vi "Control Arm Gripper.vi"() -> ()   [LabVIEW 2015]
uses:
  Global Angle.vi
panel:
  in  "last pice":dbl
  in  "last grip":dbl
  in  "y":dbl
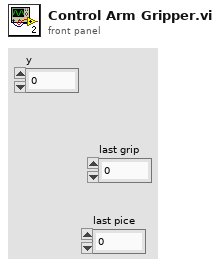
[diagram p1: front panel]
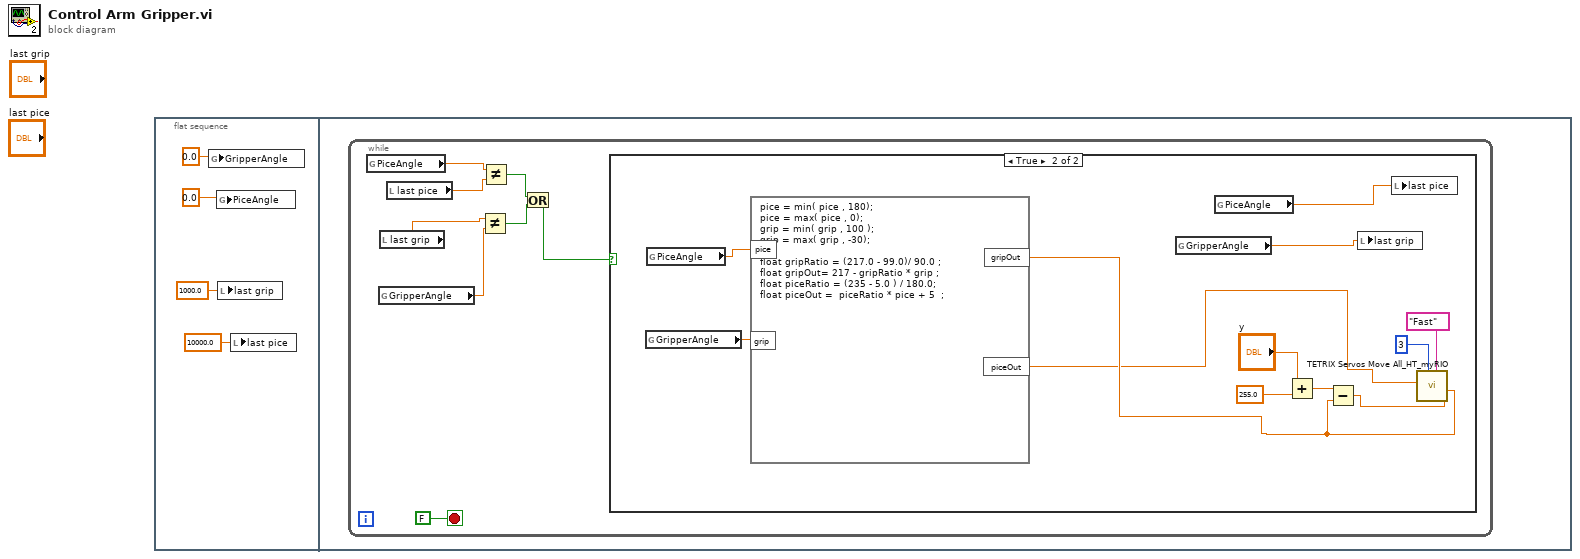
[diagram p0: block diagram]
diagram:
  n1 = flat-sequence {
    frame #0 {
      n2 = global write "Global Angle.vi" "GripperAngle"(0.0 ("GripperAngle")) -> ()
      n3 = global write "Global Angle.vi" "PiceAngle"(0.0 ("GripperAngle")) -> ()
      n4 = local write "last grip"(1000.0 ("last grip")) -> ()
      n5 = local write "last pice"(10000.0 ("last pice")) -> ()
    }
    frame #1 {
      n6 = while {
        stop <- FALSE stop-if-true
        n7 = global read "Global Angle.vi" "PiceAngle"() -> (w12:dbl)
        n8 = global read "Global Angle.vi" "GripperAngle"() -> (w9:dbl)
        n9 = local read "last grip"() -> (w10:dbl)
        n10 = local read "last pice"() -> (w11:dbl)
        n11 = Not Equal?(x=w10, y=w9) -> (x != y?=w7:bool)
        n12 = Not Equal?(x=w12, y=w11) -> (x != y?=w8:bool)
        n13 = Or(x=w8, y=w7) -> (x .or. y?=w6:bool)
        n14 = case shown="True" w6 {
          frame False {
          }
          frame True {
            n15 = global read "Global Angle.vi" "GripperAngle"() -> (w13:dbl)
            n16 = global read "Global Angle.vi" "PiceAngle"() -> (w14:dbl)
            n17 = formula code="pice = min( pice , 180);\npice = max( pice , 0);\ngrip = min( grip , 100 );\ngrip = max( grip , -30);\n\nfloat gripRatio = (217.0 - 99.0)/ 90.0 ;\nfloat gripOut= 217 - gripRatio * grip ;\nfloat piceRatio = (235 - 5.0 ) / 180.0;\nfloat piceOut =  piceRatio * pice + 5  ;"("pice"=w14, "grip"=w13) -> ("gripOut"=w16:dbl, "piceOut"=w15:dbl)
            n18 = global read "Global Angle.vi" "GripperAngle"() -> (w17:dbl)
            n19 = global read "Global Angle.vi" "PiceAngle"() -> (w18:dbl)
            n20 = Add(x=255.0, y="y") -> (x+y=w19:dbl)
            n21 = Subtract(x=w19, y=w16) -> (x-y=w23:dbl)
            n22 = local write "last grip"(w17) -> ()
            n23 = local write "last pice"(w18) -> ()
            n24 = call <vilib>:"TETRIX Servos Move All_HT_myRIO.vi"("Servo 4 (0 - 255)"=w23, "Servo 5 (0 - 255)"=w16, "Enable Sync: Fast | Medium | Slow | None"="Fast", "Controller Daisy Chain Position (1 - 4)"=u8 3, "Servo 1 (0 - 255)"=w15) -> ()  [unwired: 4 in, 1 out]
          }
        }
      }
    }
  }
